vi "Populate Case Results.vi"(8 "error in (no error)":errorcluster, 10 "Test Case Result":T1, 11 "Test Tree In":refnum<class "Test Result Tree.lvclass">) -> (0 "error out":errorcluster, 2 "Test Case Result Out out":T1, 3 "Test Tree Out":refnum<class "Test Result Tree.lvclass">)   [LabVIEW 2020, in "Test Result Tree.lvclass"]
uses:
  Framework/Helper Classes/Test Result Tree/Test Result Tree.lvclass
  C:/Git/astemes-lunit/source/Framework/Helper Classes/Test Tree/Test Tree.lvclass
  Framework/Result Types/Case Result/Test Case Result.ctl
  Framework/Result Types/Method Result/Method Result.ctl
  Result/Status.ctl
  Framework/Result Types/Assertion Result/Assertion Result.ctl
  Framework/Result Types/Assertion Result/Public/TypeDefs/Assertion Type.ctl
  Test Tree.lvclass/Test Tree.ctl
  Framework/Result Types/Case Result/Private/Merge Status.vi
  Framework/Result Types/Case Result/Test Case Result.lvlib
  Test Tree.lvclass
  Framework/Result Types/Assertion Result/Assertion Result.lvlib
  Framework/Result Types/Method Result/Method Result.lvlib
  Result/Result.lvlib
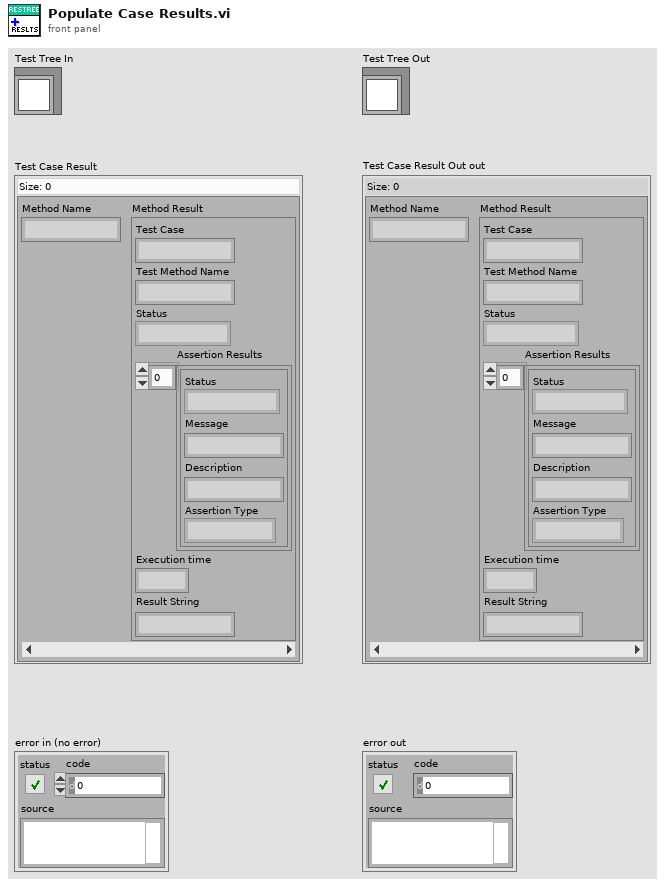
[diagram p1: front panel]
types:
  T1 = typedef "Test Case Result.lvlib/Test Case Result.ctl" = map{string, T2}
  T2 = typedef "Method Result.lvlib/Method Result.ctl" = cluster{"Test Case":string, "Test Method Name":string, "Status":T3, "Assertion Results":T4[], "Execution time":dbl, "Result String":string}
  T3 = typedef "Result.lvlib/Status.ctl" = enum16{"Passed", "Failed", "Error", "Skipped", "Setup Error", "Broken", "Teardown Error"}
  T4 = typedef "Assertion Result.lvlib/Assertion Result.ctl" = cluster{"Status":T3, "Message":string, "Description":string, "Assertion Type":T5}
  T5 = typedef "Result.lvlib/Assertion Type.ctl" = enum16{"None", "Pass", "Fail", "Skip", "Pass if Equal", "Fail if Equal", "Pass if Error", "Fail if Error", "Pass if", "Fail if"}
  T6 = map{string, cluster{"Left Cell String":string, "Child Text":string[], "Item Indent":i32, "Child Only?":bool, "Glyph Index":i32}}
  T7 = cluster{"Left Cell String":string, "Child Text":string[], "Item Indent":i32, "Child Only?":bool, "Glyph Index":i32}
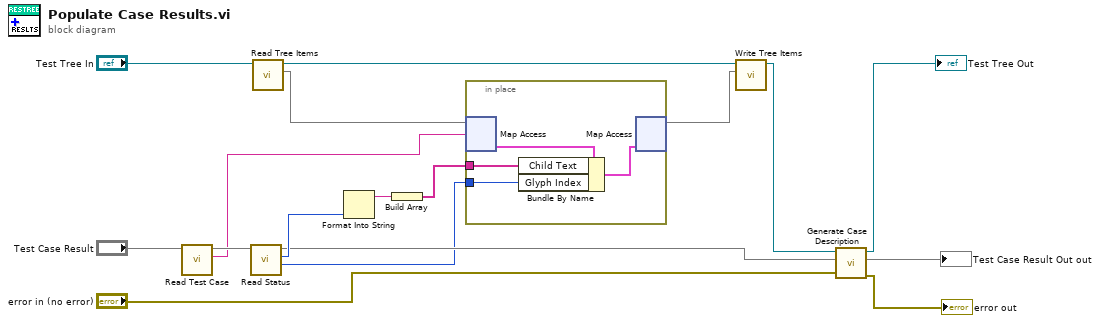
[diagram p0: block diagram]
diagram:
  n1 = call "Read Test Case.vi"("Test Case Result In"="Test Case Result") -> ("Test Case"=w7:string, "Test Case Result Out"=w16:T1)  [unwired: 9 in]
  n2 = call "Read Status.vi"("Test Case Result In"=w16) -> ("Glyph Index"=w8:i32, "Status"=w14:T3, "Test Case Result Out"=w11:T1)  [unwired: 8 in]
  n3 = call "Read Tree Items.vi"("Test Tree In"="Test Tree In") -> ("Tree Items"=w4:T6, "Test Tree Out"=w5:refnum<class "Test Result Tree.lvclass">)  [unwired: 9 in]
  n4 = Format Into String(w14) -> (resulting string=w15:string)  [unwired: 3 in, 1 out]
  n5 = Build Array(w15) -> (w9:string[])
  n6 = in-place {
    in-place-border: w9 -> [w21]
    in-place-border: w8 -> [w20]
    n7 = in-place-map #1(w4, w7) -> (w19:T7)  [unwired: 1 in, 1 out]
    n8 = Bundle By Name(cluster=w19, "Child Text"=w21, "Glyph Index"=w20) -> (w18:T7)
    n9 = in-place-map #1(w18) -> (w3:T6)  [unwired: 1 in, 2 out]
  }
  n10 = call "Write Tree Items.vi"("Tree Items"=w3, "Test Tree In"=w5) -> ("Test Tree Out"=w2:refnum<class "Test Result Tree.lvclass">)  [unwired: 9 in]
  n11 = call "Generate Case Description.vi"("error in (no error)"="error in (no error)", "Test Case Result Out in"=w11, "Test Tree In"=w2) -> ("error out"=→"error out":errorcluster, "Test Case Result Out out"=→"Test Case Result Out out":T1, "Test Tree Out"=→"Test Tree Out":refnum<class "Test Result Tree.lvclass">)  [unwired: 6 in]
